vi "TEOAE-MOCR.vi"(11 "Expt State":T5) -> ()   [LabVIEW 2015]
uses:
  CFTS Main Panel SubVIs/CFTS-Experiment State.ctl
  Typedefs/TEMOCR-Sequence Step.ctl
panel:
  in  "Run":i32
  in  "Number":i32
  in  "ID":string
  out "exit signal":bool
  in  "Sampling rate (Hz)":dbl
  in  "Save raw data?":bool
  in  "Analysis":T1
  in  "Repeats":i32
  in  "Sequence":T2
  in  "Elicitor":T3
  in  "Probe":T4
  out "Cal files":string
  out "show cal files":bool
  in  "file pattern":path
  in  "Start":bool
  in  "Stop":bool
  out "running":bool
  out "analysis":errorcluster
  out "finished":errorcluster
  out "restore defaults":bool
  out "ProgressBar":u8(slide) caption="Level: 40 Baseline" scale=0.0..500.0
  out "FreqGraph":cluster{dbl[], dbl[]}(graph)
  out "IOGraph":cluster{dbl[], dbl[]}(graph)
  out "TimeGraph":dbl[][](graph)
  # "Probe"
  # "Elicitor"
  # "Analysis"
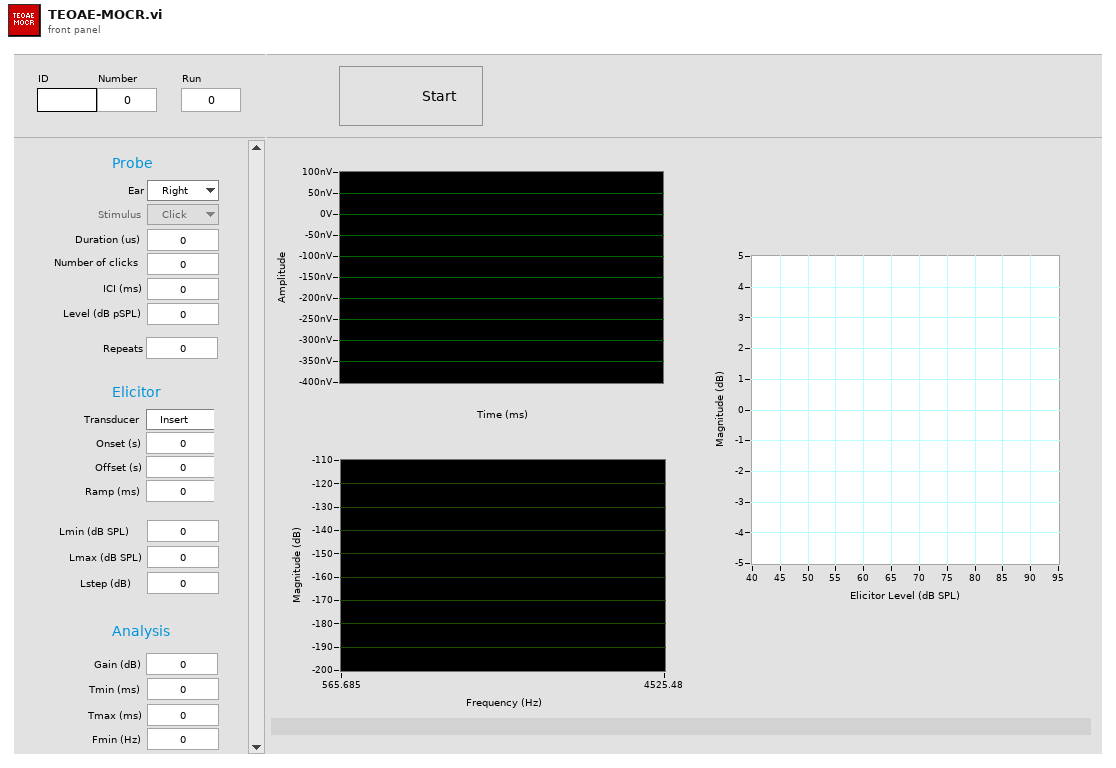
[diagram p1: front panel]
types:
  T1 = cluster{"T(ms) re peak":dbl, "T(ms) re peak 2":dbl, "Fmin (Hz)":dbl, "Fmax (Hz)":dbl, "Window":enum16{"None", "Hanning", "Hamming"}, "Highpass (Hz)":dbl, "Lowpass (Hz)":dbl, "T(ms) re peak 3":dbl}
  T2 = cluster{"Lmin (dB SPL)":dbl, "Lmax (dB SPL)":dbl, "Lstep (dB)":dbl}
  T3 = cluster{"Onset (s)":dbl, "Offset (s)":dbl, "Ramp (ms)":dbl, "Transducer":enum16{"Insert", "TDH-39", "HD300"}}
  T4 = cluster{"Ear":enum16{"Right", "Left"}, "Stimulus":enum16{"Click", "Chirp"}, "Duration (us)":dbl, "Number of clicks":dbl, "ICI (ms)":dbl, "Level (dB pSPL)":dbl}
  T5 = typedef "CFTS-Experiment State.ctl" = cluster{"Experimenter":string, "Number":u32, "Right":string, "Left":string, "Data Folder":path, "State File":path, "Version Info":string, "End Exposure Time":dbl, "Exposure Duration":string, "Run #":cluster{"CAP":i16, "ABR":i16, "DP":i16, "VsEP":i16, "MeasSeq":i16, "SubSeq":i16, "SFOAE":i16}}
  T6 = typedef "TEMOCR-IPC.ctl" = cluster{"SGDA":refnum<queue>, "AnalysisStart":refnum<queue>, "AnalysisUpdate":refnum<queue>}
  T7 = cluster{"Run":refnum<vi>, "ProgressBar":refnum<vi>, "IOGraph":refnum<vi>, "TimeGraph":refnum<vi>, "FreqGraph":refnum<vi>}
  T8 = typedef "TEMOCR-Parameters.ctl" = cluster{"Probe":T9, "Elicitor":T10, "Sequence":T12, "Analysis":T13, "Repeats":i32, "Fs (Hz)":dbl, "Cycles":i32, "save raw":bool}
  T9 = typedef "TEMOCR-Probe.ctl" = cluster{"Ear":enum16{"Right", "Left"}, "Stimulus":enum16{"Click", "Chirp"}, "Duration (us)":dbl, "Nclick":i32, "ICI (ms)":dbl, "Level":dbl}
  T10 = typedef "TEMOCR-Elicitor.ctl" = cluster{"Onset (s)":dbl, "Offset (s)":dbl, "Ramp (ms)":dbl, "Transducer":T11}
  T11 = typedef "HSTS-Transducer.ctl" = enum16{"Insert", "TDH-39", "HD300", "ER-10X"}
  T12 = typedef "TEMOCR-Sequence.ctl" = cluster{"Start":dbl, "Stop":dbl, "Step":dbl}
  T13 = typedef "TEMOCR-Analysis.ctl" = cluster{"Tmin (ms)":dbl, "Tmax (ms)":dbl, "Fmin (Hz)":dbl, "Fmax (Hz)":dbl, "Window":enum16{"None", "Hanning", "Hamming"}, "Fhp (Hz)":dbl, "Flp (Hz)":dbl, "Gain (dB)":dbl}
  T14 = typedef "TEMOCR-Sequence Step.ctl" = cluster{"Rep":i32, "Seq":i32, "Phase":i32}
  T15 = typedef "TEMOCR-AO Data.ctl" = cluster{"Pulses":dbl[], "Fs (Hz)":dbl, "Npts":i32, "mults":dbl[], "chans":i32[], "Nreps":i32, "NzeroFrames":i32, "Offset (s)":dbl, "Ramp (ms)":dbl}
  T16 = cluster{bool, "AI Waveforms":dbl[][], "Step":T14}
  T17 = typedef "TEMOCR-Analysis State.ctl" = cluster{"Data file":path, "Raw":refnum<file>, "PT":cluster{"Freq":dbl[], "Mag":dbl[]}, "IO":cluster{"Level":dbl[], "Mag":dbl[]}, "Nreps":i32, "Fs (Hz)":dbl, "Avg1":dbl[], "pts/pulse":i32, "pulses/frame":i32, "Avg2":dbl[], "Gain":dbl, "spectra":cluster{"Freq":dbl[], "Mag":dbl[][]}[]}
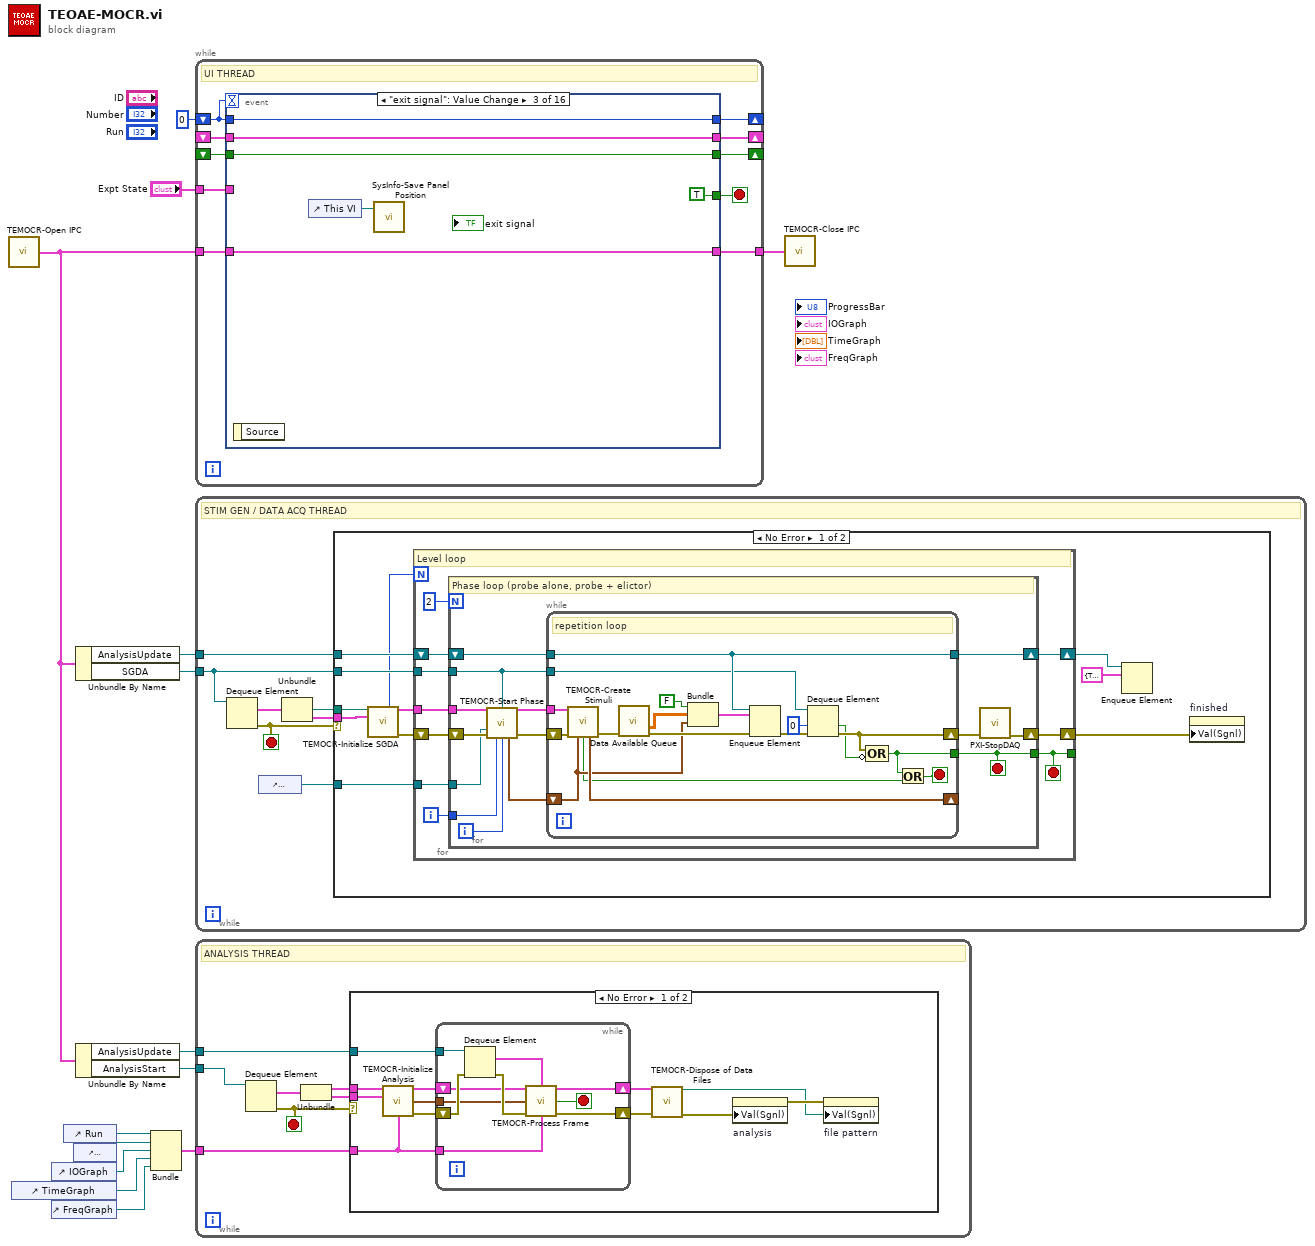
[diagram p0: block diagram]
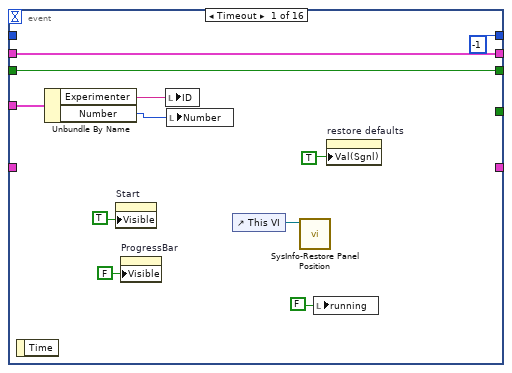
[diagram p3: hidden frame]
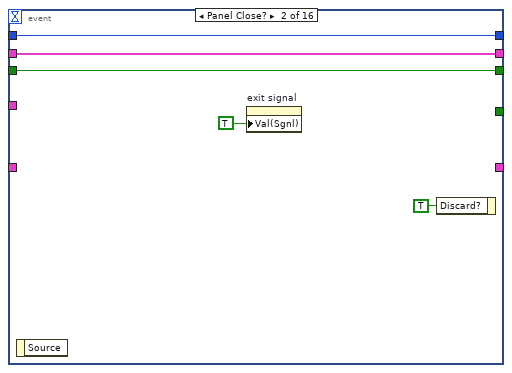
[diagram p4: hidden frame]
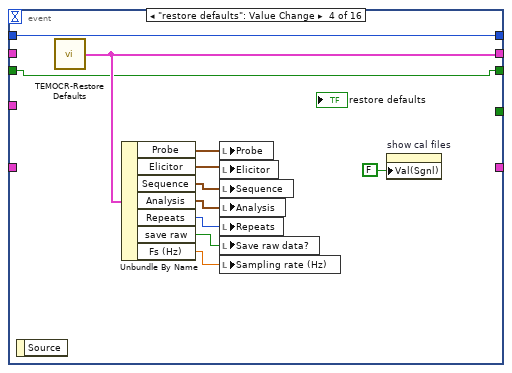
[diagram p5: hidden frame]
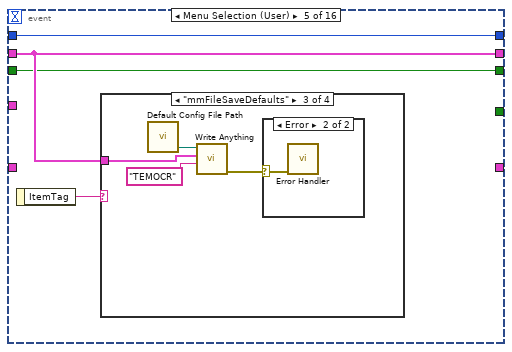
[diagram p6: hidden frame]
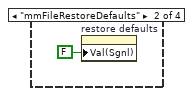
[diagram p8: hidden frame]
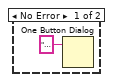
[diagram p9: hidden frame]
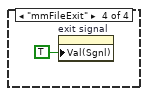
[diagram p10: hidden frame]
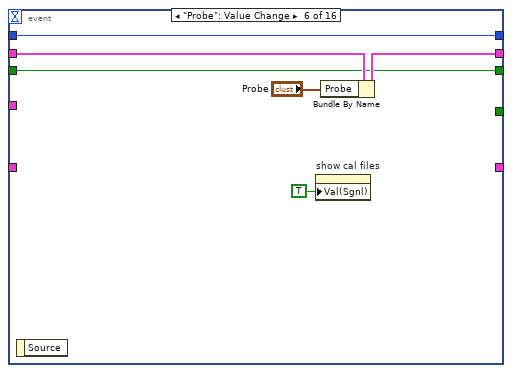
[diagram p11: hidden frame]
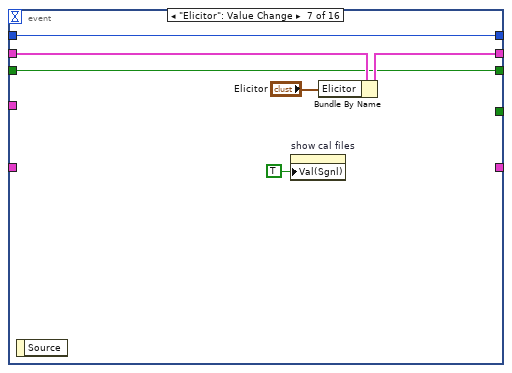
[diagram p12: hidden frame]
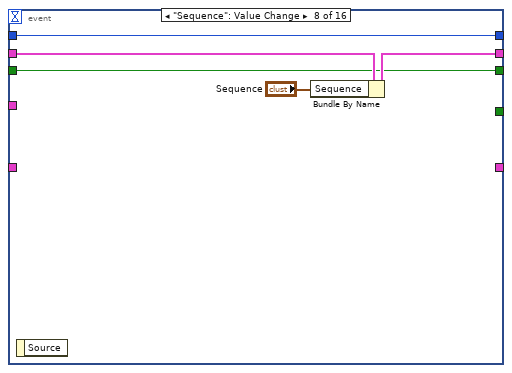
[diagram p13: hidden frame]
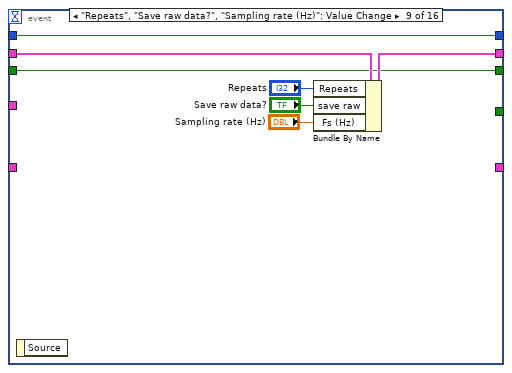
[diagram p14: hidden frame]
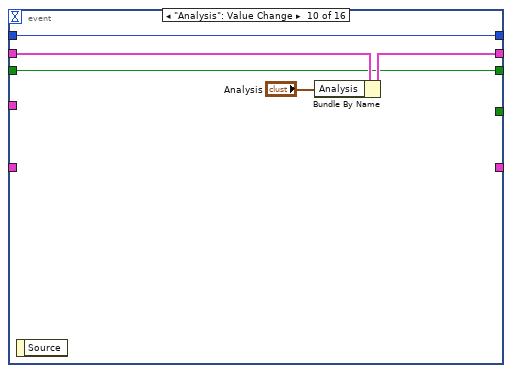
[diagram p15: hidden frame]
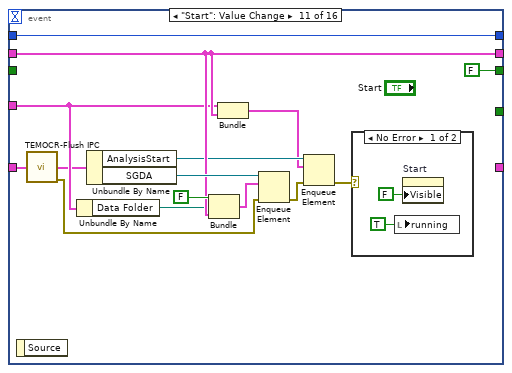
[diagram p16: hidden frame]
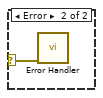
[diagram p17: hidden frame]
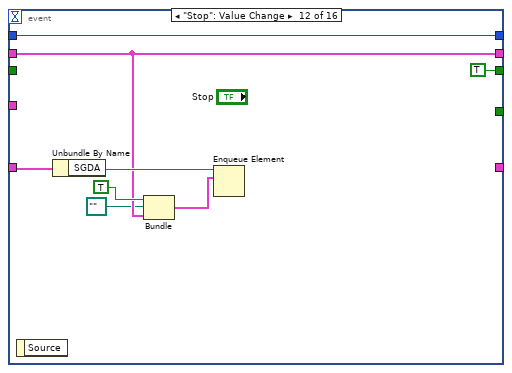
[diagram p18: hidden frame]
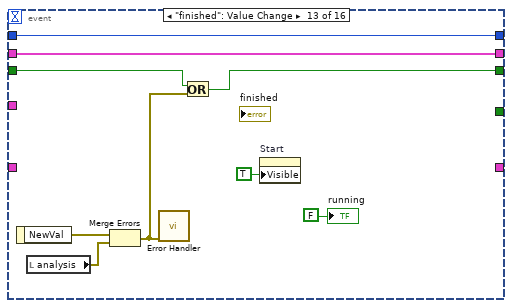
[diagram p19: hidden frame]
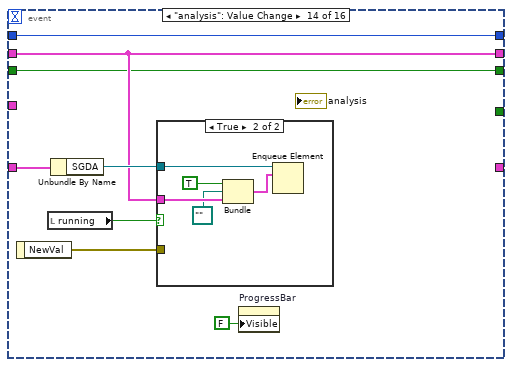
[diagram p20: hidden frame]
diagram:
  n1 = call "TEMOCR-Open IPC.vi"() -> ("IPC"=w1:T6)  [unwired: 15 in]
  n2 = control-ref of="TimeGraph"() -> (w5:refnum<vi>)
  n3 = control-ref of="IOGraph"() -> (w2:refnum<vi>)
  n4 = control-ref of="FreqGraph"() -> (w4:refnum<vi>)
  n5 = control-ref of="Run"() -> (w7:refnum<vi>)
  n6 = control-ref of="ProgressBar"() -> (w6:refnum<vi>)
  n7 = Unbundle By Name(w1) -> ("AnalysisUpdate"=w9:refnum<queue>, "SGDA"=w12:refnum<queue>)
  n8 = Unbundle By Name(w1) -> ("AnalysisUpdate"=w8:refnum<queue>, "AnalysisStart"=w11:refnum<queue>)
  n9 = Bundle("Run"=w7, "ProgressBar"=w6, "IOGraph"=w2, "TimeGraph"=w5, "FreqGraph"=w4) -> (w3:T7)  [unwired: 1 in]
  n10 = while {
    shift-right: [w23] -> _
    shift-left: 0 -> [w24]
    shift-right: [w21] -> _
    shift-left: _ -> [w20]
    tunnel: "Expt State" -> [w19]
    tunnel: w1 -> [w18]
    tunnel: [w17] -> w10
    shift-right: [w16] -> _
    shift-left: _ -> [w15]
    stop <- w22 stop-if-true
    # "UI THREAD"
    n11 = event shown="[2] \"exit signal\": Value Change" {
      selector: _ -> [_ _ _ _ _ _ _ _ _ _ _ _ _ _ _ _]
      dyn-events: _ -> [_ _ _ _ _ _ _ _ _ _ _ _ _ _ _ _]
      timeout: w24 -> [_ _ _ _ _ _ _ _ _ _ _ _ _ _ _ _]
      tunnel: w24 -> [_ w40 w46 w57 w61 w75 w81 w86 w93 w98 w113 w124 w133 w141 w152 w183]
      tunnel: [-1 w40 w46 w57 w61 w75 w81 w86 w93 w98 w113 w124 w133 w141 w152 w183] -> w23
      tunnel: [_ _ TRUE _ _ _ _ _ _ _ _ _ _ _ _ _] -> w22
      tunnel: [w33 w37 w44 w56 w59 w73 w79 w84 w91 w96 w109 w119 w132 w137 w151 w169] -> w21
      tunnel: w20 -> [w33 w37 w44 _ w59 w74 w80 w85 w92 w97 w109 w119 w132 w137 w151 w169]
      tunnel: w19 -> [w31 _ _ _ _ _ _ _ _ _ w104 _ _ _ _ w168]
      tunnel: w18 -> [_ _ w42 _ _ _ _ _ _ _ w102 w123 _ w139 _ _]
      tunnel: [_ _ w42 _ _ _ _ _ _ _ _ _ _ _ _ _] -> w17
      tunnel: [w25 w36 w41 w48 w58 w71 w77 w82 w87 w94 FALSE ("file query") TRUE w125 w135 w149 w182] -> w16
      tunnel: w15 -> [w25 w36 w41 w48 w58 w71 w77 w82 w87 w94 _ _ w126 w135 w149 w182]
      event Timeout {
        n12 = event-data() -> ()  [unwired: 1 in, 1 out]
        n13 = Unbundle By Name(w31) -> ("Experimenter"=w30:string, "Number"=w29:u32)
        n14 = property on="Start" class="Bool"("Visible"=TRUE) -> ()  [unwired: 2 in, 2 out]
        n15 = property on="ProgressBar" class="Slide (strict)"("Visible"=FALSE) -> ()  [unwired: 2 in, 2 out]
        n16 = local write "ID"(w30) -> ()
        n17 = local write "Number"(w29) -> ()
        n18 = control-ref of="This VI"() -> (w32:refnum<vi>)
        n19 = call "SysInfo-Restore Panel Position.vi"("VI Refnum"=w32) -> ()  [unwired: 12 in, 3 out]
        n20 = local write "running"(FALSE ("running")) -> ()
        n21 = property on="restore defaults" class="Bool (strict)"("Val(Sgnl)"=TRUE ("Value (Signaling)")) -> ()  [unwired: 2 in, 2 out]
      }
      event Panel Close? {
        n22 = event-data() -> ()  [unwired: 1 in, 1 out]
        n23 = property on="exit signal" class="Bool (strict)"("Val(Sgnl)"=TRUE ("Value (Signaling)")) -> ()  [unwired: 2 in, 2 out]
        n24 = event-data("Discard?"=TRUE) -> ()  [unwired: 1 in, 1 out]
      }
      event "exit signal": Value Change {
        n25 = event-data() -> ()  [unwired: 1 in, 1 out]
        n26 = control-ref of="This VI"() -> (w43:refnum<vi>)
        n27 = call "SysInfo-Save Panel Position.vi"("VI Refnum"=w43) -> ()  [unwired: 14 in, 1 out]
      }
      event "restore defaults": Value Change {
        n28 = event-data() -> ()  [unwired: 1 in, 1 out]
        n29 = call "TEMOCR-Restore Defaults.vi"() -> ("Params"=w56:T8)  [unwired: 15 in]
        n30 = Unbundle By Name(w56) -> ("Probe"=w55:T9, "Elicitor"=w54:T10, "Sequence"=w53:T12, "Analysis"=w52:T13, "Repeats"=w51:i32, "save raw"=w50:bool, "Fs (Hz)"=w49:dbl)
        n31 = local write "Probe"(w55) -> ()
        n32 = local write "Elicitor"(w54) -> ()
        n33 = local write "Sequence"(w53) -> ()
        n34 = local write "Analysis"(w52) -> ()
        n35 = local write "Repeats"(w51) -> ()
        n36 = local write "Save raw data?"(w50) -> ()
        n37 = local write "Sampling rate (Hz)"(w49) -> ()
        n38 = property on="show cal files" class="Bool (strict)"("Val(Sgnl)"=FALSE ("Value (Signaling)")) -> ()  [unwired: 2 in, 2 out]
      }
      event Menu Selection (User) {
        n39 = event-data() -> ("ItemTag"=w60:string)  [unwired: 1 in]
        n40 = case shown="\"mmFileSaveDefaults\"" w60 {
          tunnel: w59 -> [_ _ w65 _]
          frame "False", Default {
          }
          frame "mmFileRestoreDefaults" {
            n41 = property on="restore defaults" class="Bool (strict)"("Val(Sgnl)"=FALSE ("Value (Signaling)")) -> ()  [unwired: 2 in, 2 out]
          }
          frame "mmFileSaveDefaults" {
            n42 = call "Default Config File Path.vi"() -> ("Default config file name"=w66:path)
            n43 = call "Write Anything.vi"("Section Name (Name of \"Anything\")"="TEMOCR" ("Section Name (Name of \"Anything\")"), "Anything"=w65, "Path (dialog)"=w66) -> ("Error Out"=w63:errorcluster)  [unwired: 7 in, 1 out]
            n44 = case shown="Error" w63 {
              selector: w63 -> [_ w68]
              frame No Error {
                n45 = One Button Dialog(message="Defaults saved.") -> ()  [unwired: 1 in, 1 out]
              }
              frame Error {
                n46 = call "Error Handler.vi"("error in (no error)"=w68) -> ()  [unwired: 13 in, 2 out]
              }
            }
          }
          frame "mmFileExit" {
            n47 = property on="exit signal" class="Bool (strict)"("Val(Sgnl)"=TRUE ("Value (Signaling)")) -> ()  [unwired: 2 in, 2 out]
          }
        }
      }
      event "Probe": Value Change {
        n48 = event-data() -> ()  [unwired: 1 in, 1 out]
        n49 = property on="show cal files" class="Bool (strict)"("Val(Sgnl)"=TRUE ("Value (Signaling)")) -> ()  [unwired: 2 in, 2 out]
        n50 = Bundle By Name(cluster=w74, "Probe"="Probe") -> (w73:T8)
      }
      event "Elicitor": Value Change {
        n51 = event-data() -> ()  [unwired: 1 in, 1 out]
        n52 = property on="show cal files" class="Bool (strict)"("Val(Sgnl)"=TRUE ("Value (Signaling)")) -> ()  [unwired: 2 in, 2 out]
        n53 = Bundle By Name(cluster=w80, "Elicitor"="Elicitor") -> (w79:T8)
      }
      event "Sequence": Value Change {
        n54 = event-data() -> ()  [unwired: 1 in, 1 out]
        n55 = Bundle By Name(cluster=w85, "Sequence"="Sequence") -> (w84:T8)
      }
      event "Repeats", "Save raw data?", "Sampling rate (Hz)": Value Change {
        n56 = event-data() -> ()  [unwired: 1 in, 1 out]
        n57 = Bundle By Name(cluster=w92, "Repeats"="Repeats", "save raw"="Save raw data?", "Fs (Hz)"="Sampling rate (Hz)") -> (w91:T8)
      }
      event "Analysis": Value Change {
        n58 = event-data() -> ()  [unwired: 1 in, 1 out]
        n59 = Bundle By Name(cluster=w97, "Analysis"="Analysis") -> (w96:T8)
      }
      event "Start": Value Change {
        n60 = event-data() -> ()  [unwired: 1 in, 1 out]
        n61 = call "TEMOCR-Flush IPC.vi"("IPC"=w102) -> ("IPC thru"=w101:T6, "error out"=w100:errorcluster)  [unwired: 13 in]
        n62 = Unbundle By Name(w104) -> ("Data Folder"=w103:path)
        n63 = Unbundle By Name(w101) -> ("AnalysisStart"=w108:refnum<queue>, "SGDA"=w112:refnum<queue>)
        n64 = Bundle(FALSE, "Data Folder"=w103, "Params"=w109) -> (w110:cluster{bool, "Data Folder":path, "Params":T8})  [unwired: 1 in]
        n65 = Bundle("Expt State"=w104, "Params"=w109) -> (w107:cluster{"Expt State":T5, "Params":T8})  [unwired: 1 in]
        n66 = Enqueue Element(queue=w112, element=w110, error in (no error)=w100) -> (error out=w106:errorcluster)  [unwired: 1 in, 2 out]
        n67 = Enqueue Element(queue=w108, element=w107, error in (no error)=w106) -> (error out=w105:errorcluster)  [unwired: 1 in, 2 out]
        n68 = case shown="No Error" w105 {
          selector: w105 -> [_ w116]
          frame No Error {
            n69 = local write "running"(TRUE ("running")) -> ()
            n70 = property on="Start" class="Bool"("Visible"=FALSE) -> ()  [unwired: 2 in, 2 out]
          }
          frame Error {
            n71 = call "Error Handler.vi"("error in (no error)"=w116) -> ()  [unwired: 13 in, 2 out]
          }
        }
      }
      event "Stop": Value Change {
        n72 = event-data() -> ()  [unwired: 1 in, 1 out]
        n73 = Unbundle By Name(w123) -> ("SGDA"=w121:refnum<queue>)
        n74 = Bundle(TRUE, path "", "Params"=w119) -> (w120:cluster{bool, path, "Params":T8})  [unwired: 1 in]
        n75 = Enqueue Element(queue=w121, element=w120) -> ()  [unwired: 2 in, 3 out]
      }
      event "finished": Value Change {
        n76 = event-data() -> ("NewVal"=w129:errorcluster)  [unwired: 1 in]
        n77 = local read "analysis"() -> (w128:errorcluster)
        n78 = Merge Errors(w129, w128) -> (w127:errorcluster)
        n79 = call "Error Handler.vi"("error in (no error)"=w127) -> ()  [unwired: 13 in, 2 out]
        n80 = Or(x=w126, y=w127) -> (x .or. y?=w125:bool)
        n81 = property on="Start" class="Bool"("Visible"=TRUE) -> ()  [unwired: 2 in, 2 out]
        "running" <- FALSE ("running")
      }
      event "analysis": Value Change {
        n82 = event-data() -> ("NewVal"=w136:errorcluster)  [unwired: 1 in]
        n83 = local read "running"() -> (w140:bool)
        n84 = Unbundle By Name(w139) -> ("SGDA"=w138:refnum<queue>)
        n85 = case shown="True" w140 {
          tunnel: w138 -> [_ w147]
          tunnel: w137 -> [_ w146]
          tunnel: w136 -> [w142 _]
          frame False {
            n86 = call "Error Handler.vi"("error in (no error)"=w142) -> ()  [unwired: 13 in, 2 out]
          }
          frame True {
            n87 = Bundle(TRUE, path "", "Params"=w146) -> (w143:cluster{bool, path, "Params":T8})  [unwired: 1 in]
            n88 = Enqueue Element(queue=w147, element=w143) -> ()  [unwired: 2 in, 3 out]
          }
        }
        n89 = property on="ProgressBar" class="Slide (strict)"("Visible"=FALSE) -> ()  [unwired: 2 in, 2 out]
      }
      event "file pattern": Value Change {
        n90 = event-data() -> ()  [unwired: 1 in, 1 out]
        n91 = case shown="True" w149 {
          tunnel: [TRUE ("T button?") w154] -> w148
          frame False {
          }
          frame True {
            n92 = Two Button Dialog(message="Data collection aborted.\nSave last file?", 1:"No" ("F button name (\"Cancel\")"), 2:"Yes" ("T button name (\"OK\")")) -> (T button?=w154:bool)
          }
        }
        n93 = case shown="False" w148 {
          tunnel: "file pattern" -> [w162 _]
          frame False {
            n94 = Strip Path(path=w162) -> (stripped path=w161:path, name=w160:string)
            n95 = List Folder(path=w161, pattern=w160) -> (path out=w159:path, filenames=w158:string[])  [unwired: 2 in, 2 out]
            n96 = for {
              tunnel: w159 -> [w166]
              tunnel: w158 -> [w165] mode=indexing
              tunnel: [w163] -> _
              n97 = Build Path(base path=w166, name or relative path=w165) -> (appended path=w164:path)
              n98 = Delete(path (use dialog)=w164) -> (error out=w163:errorcluster)  [unwired: 4 in, 2 out]
            }
          }
          frame True {
          }
        }
      }
      event "show cal files": Value Change {
        n99 = event-data() -> ()  [unwired: 1 in, 1 out]
        n100 = Unbundle By Name(w169) -> ("Elicitor.Transducer"=w175:T11)
        n101 = Unbundle By Name(w169) -> ("Probe.Ear"=w172:enum16{"Right", "Left"})
        n102 = Unbundle By Name(w168) -> ("Data Folder"=w173:path)
        n103 = case shown="\"Right\"" w172 {
          tunnel: ["Left" "Right"] -> w171
          tunnel: ["Right" "Left"] -> w174
          frame "Left" {
          }
          frame "Right" {
          }
        }
        n104 = Format Into String(w175) -> (resulting string=w176:string)  [unwired: 3 in, 1 out]
        n105 = call "HSTS-Calibration Path.vi"("Data Folder"=w173, "Speaker"="ER10X", "Side"=w171) -> ("Cal Path"=w177:path)  [unwired: 11 in, 1 out]
        n106 = call "HSTS-Calibration Path.vi"("Data Folder"=w173, "Speaker"=w176, "Side"=w174) -> ("Cal Path"=w178:path)  [unwired: 11 in, 1 out]
        n107 = Path To String(path=w177) -> (string=w180:string)
        n108 = Path To String(path=w178) -> (string=w181:string)
        n109 = property on="Ear" class="Enum (strict)"("TipStrip"=w180) -> ()  [unwired: 2 in, 2 out]
        n110 = Format Into String(format string="%s; %s", w180, w181) -> (resulting string=→"Cal files":string)  [unwired: 2 in, 1 out]
        n111 = property on="Transducer" class="Enum (strict)"("TipStrip"=w181) -> ()  [unwired: 2 in, 2 out]
      }
    }
  }
  n112 = while {
    tunnel: w12 -> [w189]
    tunnel: w9 -> [w190]
    stop <- w193 stop-if-true
    # "STIM GEN / DATA ACQ THREAD"
    n113 = Dequeue Element(queue=w189) -> (element=w194:cluster{bool, path, "Params":T8}, error out=w193:errorcluster)  [unwired: 2 in, 2 out]
    n114 = control-ref of="ProgressBar"() -> (w188:refnum<vi>)
    n115 = Unbundle(w194) -> (w192:path, "Params"=w191:T8)  [unwired: 1 out]
    n116 = case shown="No Error" w193 {
      tunnel: w192 -> [w205 _]
      tunnel: w191 -> [w204 _]
      tunnel: w190 -> [w202 _]
      tunnel: w189 -> [w201 _]
      tunnel: w188 -> [w197 _]
      frame No Error {
        n117 = call "TEMOCR-Initialize SGDA.vi"("Data folder"=w205, "Params"=w204) -> ("Num Levels"=w196:i32, "AO"=w203:T15, "error out"=w198:errorcluster)  [unwired: 11 in]
        n118 = for {
          N: w196 -> [_]
          tunnel: w203 -> [w215]
          tunnel: w201 -> [w213]
          shift-right: [w211] -> w200
          shift-left: w202 -> [w214]
          shift-right: [w212] -> w195
          shift-left: w198 -> [w210]
          tunnel: w197 -> [w207]
          tunnel: [w206] -> _
          i -> [w208]
          stop <- w206 stop-if-true
          # "Level loop"
          n119 = for {
            N: 2 -> [_]
            tunnel: w215 -> [w222]
            tunnel: w213 -> [w221]
            shift-right: [w228] -> w211
            shift-left: w214 -> [w229]
            shift-right: [w226] -> w212
            shift-left: w210 -> [w225]
            tunnel: w208 -> [w217]
            tunnel: w207 -> [w219]
            tunnel: [w216] -> w206
            i -> [w218]
            stop <- w216 stop-if-true
            # "Phase loop (probe alone, probe + elictor)"
            n120 = call "TEMOCR-Start Phase.vi"("AO in"=w222, "SGDA Queue"=w221, "ProgressBar"=w219, "error in (no error)"=w225, "seqStep"=w217, "phase"=w218) -> ("AO out"=w224:T15, "Step"=w220:T14, "error out"=w223:errorcluster)  [unwired: 7 in]
            n121 = while {
              tunnel: w224 -> [w247]
              tunnel: w229 -> [w237]
              shift-right: [w238] -> w227
              shift-left: w223 -> [w246]
              shift-right: [w242] -> _
              shift-left: w220 -> [w236]
              tunnel: w221 -> [w230]
              tunnel: [w237] -> w228
              tunnel: [w233] -> w216
              stop <- w232 stop-if-true
              # "repetition loop"
              n122 = call "TEMOCR-Create Stimuli.vi"("AO"=w247, "error in (no error)"=w246, "Step In"=w236) -> ("finished"=w231:bool, "Step"=w242:T14, "error out"=w245:errorcluster)  [unwired: 10 in]
              n123 = call "Data Available Queue.vi"("error in (no error)"=w245) -> ("AI Waveforms"=w243:dbl[][], "error out"=w244:errorcluster)  [unwired: 10 in, 3 out]
              n124 = Bundle(FALSE, "AI Waveforms"=w243, "Step"=w236) -> (w240:T16)  [unwired: 1 in]
              n125 = Enqueue Element(queue=w237, element=w240, error in (no error)=w244) -> (error out=w239:errorcluster)  [unwired: 1 in, 2 out]
              n126 = Dequeue Element(queue=w230, timeout in ms (-1)=0, error in (no error)=w239) -> (timed out?=w234:bool, error out=w238:errorcluster)  [unwired: 2 out]
              n127 = Compound Arithmetic op=OR(w238, invert w234) -> (w233:bool)
              n128 = Or(x=w233, y=w231) -> (x .or. y?=w232:bool)
            }
            n129 = call "PXI-StopDAQ.vi"("error in (no error)"=w227) -> ("error out"=w226:errorcluster)  [unwired: 6 in]
          }
        }
        n130 = Enqueue Element(queue=w200, element=cluster{bool, dbl[][], "Sequence":T14} {TRUE, [], "Sequence"={"Rep"=0, "Seq"=0, "Phase"=0}}) -> ()  [unwired: 2 in, 3 out]
        n131 = property on="finished" class="Clust (strict)"("Val(Sgnl)"=w195) -> ()  [unwired: 2 in, 2 out]
      }
      frame Error {
      }
    }
  }
  n132 = while {
    tunnel: w11 -> [w253]
    tunnel: w8 -> [w251]
    tunnel: w3 -> [w250]
    stop <- w252 stop-if-true
    # "ANALYSIS THREAD"
    n133 = Dequeue Element(queue=w253) -> (element=w254:cluster{"Expt State":T5, "Params":T8}, error out=w252:errorcluster)  [unwired: 2 in, 2 out]
    n134 = Unbundle(w254) -> ("Expt State"=w249:T5, "Params"=w248:T8)
    n135 = case shown="No Error" w252 {
      tunnel: w251 -> [w265 _]
      tunnel: w250 -> [w261 _]
      tunnel: w249 -> [w266 _]
      tunnel: w248 -> [w255 _]
      frame No Error {
        n136 = call "TEMOCR-Initialize Analysis.vi"("Expt State"=w266, "Params"=w255, "controls"=w261) -> ("State"=w264:T17, "Analysis"=w263:T13, "error out"=w262:errorcluster)  [unwired: 10 in]
        n137 = while {
          tunnel: w265 -> [w275]
          tunnel: w263 -> [w271]
          shift-right: [w273] -> w260
          shift-left: w262 -> [w276]
          tunnel: w261 -> [w270]
          shift-right: [w268] -> w259
          shift-left: w264 -> [w272]
          stop <- w269 stop-if-true
          n138 = Dequeue Element(queue=w275, error in (no error)=w276) -> (element=w267:cluster{bool, dbl[][], "Sequence":T14}, error out=w274:errorcluster)  [unwired: 1 in, 2 out]
          n139 = call "TEMOCR-Process Frame.vi"("State In"=w272, "queue data"=w267, "Analysis"=w271, "error in (no error)"=w274, "controls"=w270) -> ("State Out"=w268:T17, "finished"=w269:bool, "error out"=w273:errorcluster)  [unwired: 8 in]
        }
        n140 = call "TEMOCR-Dispose of Data Files.vi"("State"=w259, "error in (no error)"=w260) -> ("file pattern"=w256:path, "error out"=w258:errorcluster)  [unwired: 12 in]
        n141 = property on="analysis" class="Clust (strict)"("Val(Sgnl)"=w258) -> (error out=w257:errorcluster)  [unwired: 2 in, 1 out]
        n142 = property on="file pattern" class="Path"(error in=w257, "Val(Sgnl)"=w256) -> ()  [unwired: 1 in, 2 out]
      }
      frame Error {
      }
    }
  }
  n143 = call "TEMOCR-Close IPC.vi"("IPC"=w10) -> ()  [unwired: 15 in]
